vi "tearDown.vi"(8 "error in (no error)":errorcluster, 11 "reference in":refnum<class "Common System Tests.lvclass">) -> (0 "error out":errorcluster, 3 "reference out":refnum<class "Common System Tests.lvclass">)   [LabVIEW 2019, in "Common System Tests.lvclass"]
doc: "tearDown runs after the test method has completed. Use this method to clean up any operations or references that were opened by setUp or the test method. Unit tests should be independent of other unit tests so this VI should ensure that the next test can run in a 'clean' test environment."
uses:
  Common System Tests.lvclass
  Assets/TCP_Listener.vi
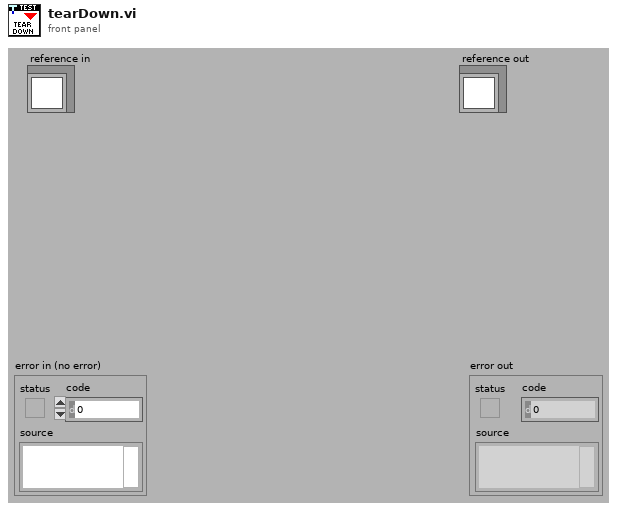
[diagram p1: front panel]
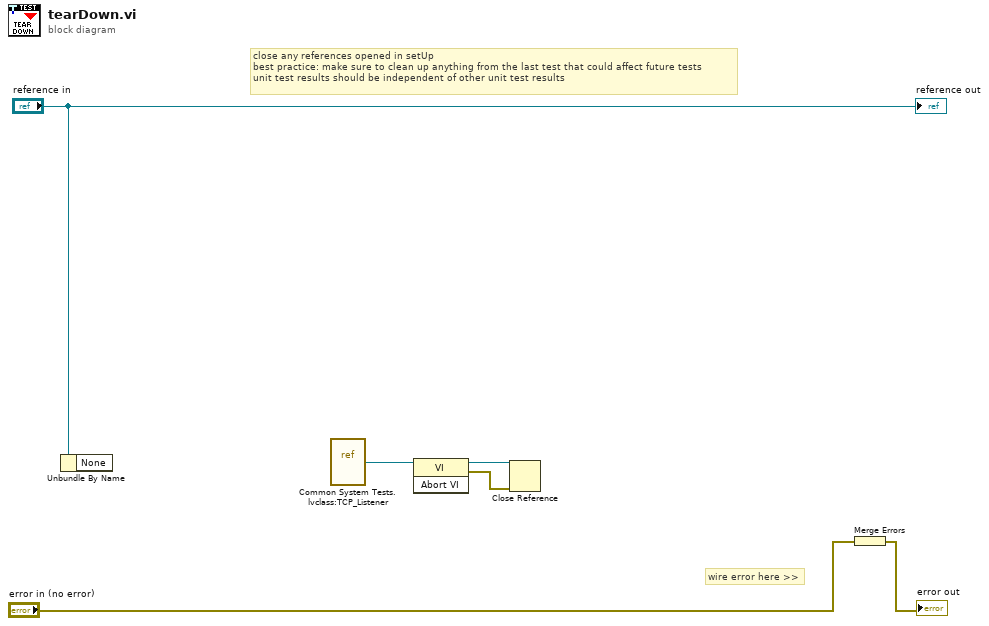
[diagram p0: block diagram]
diagram:
  # "wire error here >>"
  # "close any references opened in setUp\nbest practice: make sure to clean up anything from the last test that could affect future tests\nunit test results should be independent of other unit test results"
  n1 = Unbundle By Name("reference in") -> ()  [unwired: 1 out]
  n2 = vi-ref "Common System Tests.lvclass:TCP_Listener.vi"() -> (w4:refnum<vi>)
  n3 = invoke class="VI" method="Abort VI"(reference=w4) -> (reference out=w2:refnum<vi>, error out=w1:errorcluster)  [unwired: 2 in, 1 out]
  n4 = Close Reference(reference=w2, error in (no error)=w1) -> ()  [unwired: 1 out]
  n5 = Merge Errors("error in (no error)") -> (→"error out":errorcluster)
  "reference out" <- "reference in"
